vi "Wait for Connection.vi"(8 "error in (no error)":errorcluster, 9 "Timeout S (30)":dbl=30.0, 11 "FormulaG API in":refnum<class "FormulaG API.lvclass">) -> (0 "error out":errorcluster, 3 "FormulaG API out":refnum<class "FormulaG API.lvclass">, 4 "Time":dbl)   [LabVIEW 2020, in "FormulaG.lvlib" / "FormulaG API.lvclass"]
uses:
  FormulaG API.lvclass
  FormulaG API.lvclass/FormulaG API.ctl
  <vilib>/IlluminatedG/IG GodotServer/GodotLV/GodotServer/GodotServer.lvclass
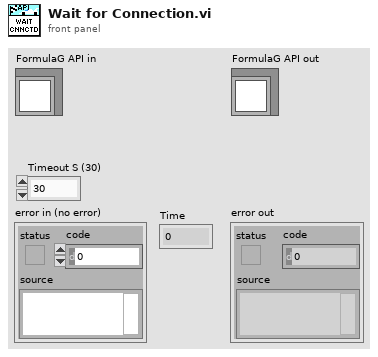
[diagram p1: front panel]
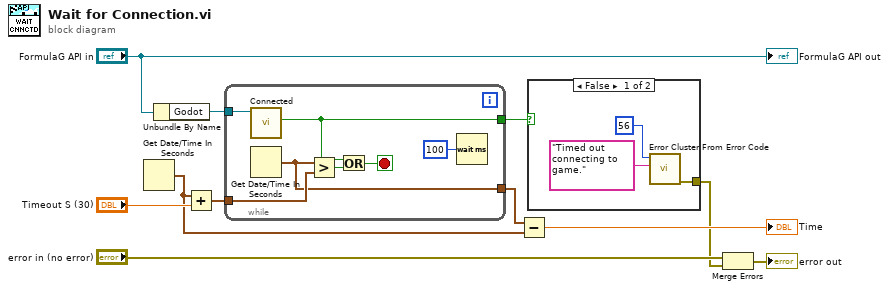
[diagram p0: block diagram]
diagram:
  n1 = Get Date/Time In Seconds() -> (seconds since 1Jan1904=w5:timestamp)
  n2 = Unbundle By Name("FormulaG API in") -> ("Godot"=w9:refnum<class "GodotServer.lvclass">)
  n3 = Add(x=w5, y="Timeout S (30)") -> (x+y=w6:timestamp)
  n4 = while {
    tunnel: w9 -> [w18]
    tunnel: w6 -> [w17]
    tunnel: [w15] -> w3
    tunnel: [w12] -> w7
    stop <- w14 stop-if-true
    n5 = call <vilib>:"Connected.vi"("GodotServer in"=w18) -> ("Connected"=w15:bool)  [unwired: 8 in, 2 out]
    n6 = Get Date/Time In Seconds() -> (seconds since 1Jan1904=w12:timestamp)
    n7 = Greater?(x=w12, y=w17) -> (0:w16:bool)
    n8 = Or(x=w15, y=w16) -> (x .or. y?=w14:bool)
    n9 = Wait (ms)(milliseconds to wait=u32 100) -> ()  [unwired: 1 out]
  }
  n10 = Subtract(x=w7, y=w5) -> (x-y=→"Time":dbl)
  n11 = case shown="False" w3 {
    tunnel: [w19 _] -> w1
    frame False {
      n12 = call <vilib>:"Error Cluster From Error Code.vi"("error message (\"\")"="Timed out connecting to game." ("error message (\"\")"), "error code (0)"=56) -> ("error out"=w19:errorcluster)  [unwired: 7 in]
    }
    frame True {
    }
  }
  n13 = Merge Errors("error in (no error)", w1) -> (→"error out":errorcluster)
  "FormulaG API out" <- "FormulaG API in"
